vi "distance.vi"(4 "y2":dbl, 6 "x2":dbl, 8 "y1":dbl, 9 "x1":dbl, 10 "子数组 2":dbl[](array[numeric]), 11 "子数组":dbl[](array[numeric])) -> (0 "distancex1x2y1y2":dbl, 3 "distance":dbl)   [LabVIEW 2014]
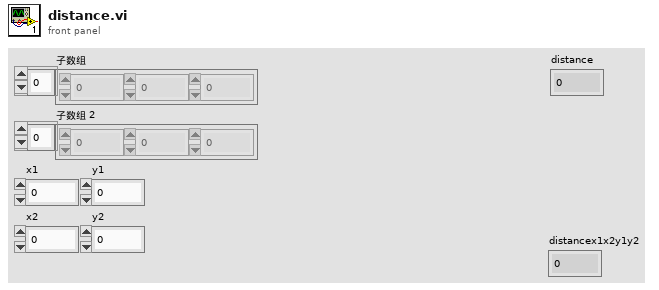
[diagram p1: front panel]
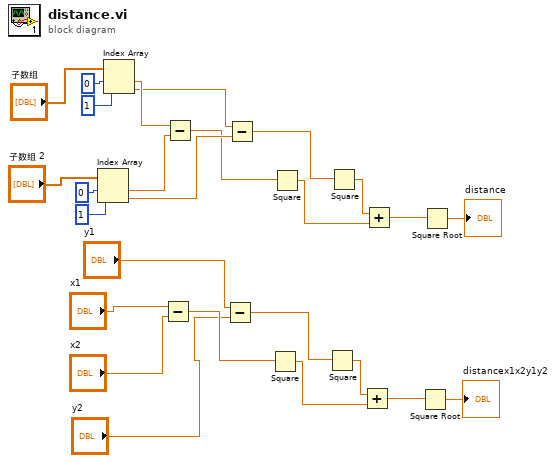
[diagram p0: block diagram]
diagram:
  n1 = Index Array(array="子数组 2", index #1=0 ("索引"), index #2=1 ("索引")) -> (element #1=w19:dbl, element #2=w17:dbl)
  n2 = Index Array(array="子数组", index #1=0 ("索引"), index #2=1 ("索引")) -> (element #1=w20:dbl, element #2=w18:dbl)
  n3 = Subtract(x="x1", y="x2") -> (x-y=w5:dbl)
  n4 = Subtract(x=w20, y=w19) -> (x-y=w16:dbl)
  n5 = Subtract(x="y1", y="y2") -> (x-y=w6:dbl)
  n6 = Subtract(x=w18, y=w17) -> (x-y=w15:dbl)
  n7 = Square(x=w5) -> (x^2=w8:dbl)
  n8 = Square(x=w16) -> (x^2=w13:dbl)
  n9 = Square(x=w6) -> (x^2=w7:dbl)
  n10 = Square(x=w15) -> (x^2=w14:dbl)
  n11 = Add(x=w7, y=w8) -> (x+y=w9:dbl)
  n12 = Add(x=w14, y=w13) -> (x+y=w12:dbl)
  n13 = Square Root(x=w9) -> (sqrt(x)=→"distancex1x2y1y2":dbl)
  n14 = Square Root(x=w12) -> (sqrt(x)=→"distance":dbl)
